vi "GEM_BANK_Add_Data.vi"(8 "error in (no error)":errorcluster, 10 "GEM_DATA":T1, 11 "LVBANK in":refnum<class "GEM_BANK.lvclass">) -> (0 "error out":errorcluster, 2 "Bank Size (bytes)":u32, 3 "LVBANK out":refnum<class "GEM_BANK.lvclass">)   [LabVIEW 2018, in "GEM_BANK.lvclass"]
uses:
  GEM_BANK.lvclass
  GEM_DATA_cluster_typedef.ctl
  GEM_BANK.lvclass/GEM_BANK.ctl
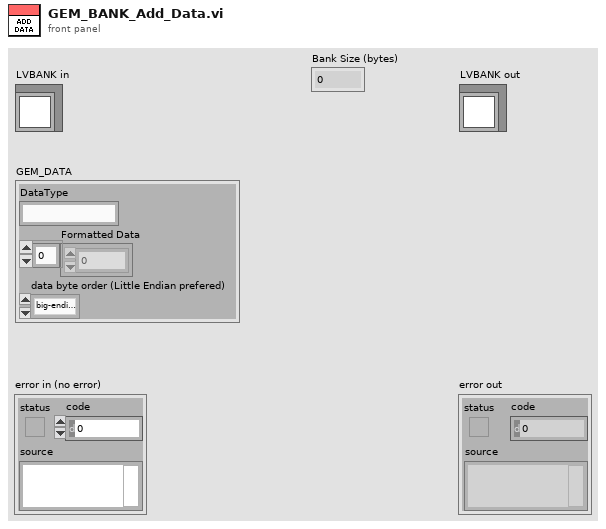
[diagram p1: front panel]
types:
  T1 = typedef "GEM_DATA_cluster_typedef.ctl" = cluster{"DataType":string, "Formatted Data":u8[], "data byte order (Little Endian prefered)":enum16{"big-endian, network order", "native, host order", "little-endian"}}
  T2 = enum16{"big-endian, network order", "native, host order", "little-endian"}
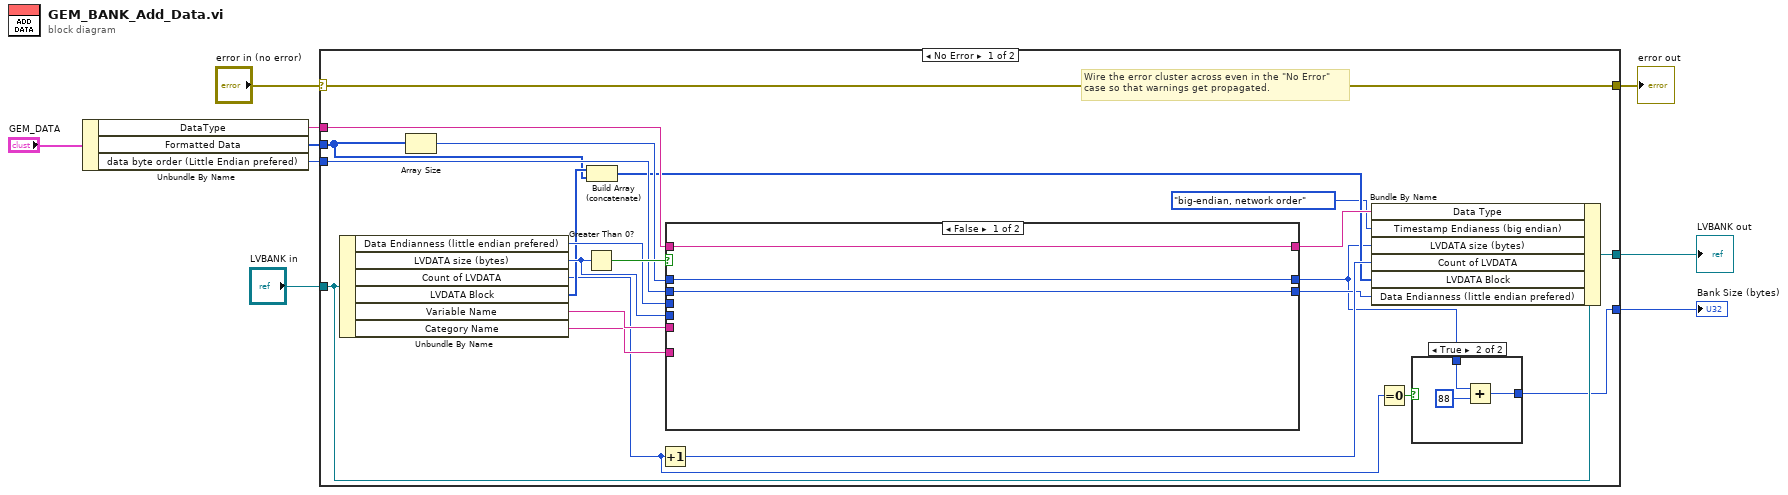
[diagram p0: block diagram]
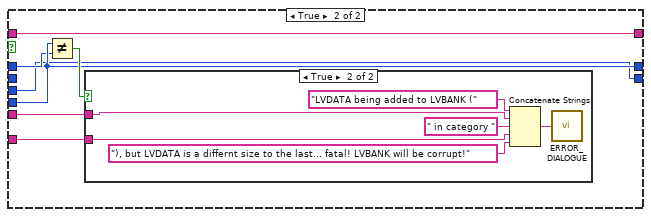
[diagram p3: hidden frame]
diagram:
  n1 = Unbundle By Name("GEM_DATA") -> ("DataType"=w3:string, "Formatted Data"=w4:u8[], "data byte order (Little Endian prefered)"=w2:T2)
  n2 = case shown="No Error" "error in (no error)" {
    selector: "error in (no error)" -> [w31 w53]
    tunnel: [w31 w53] -> w8
    tunnel: [w29 w52] -> w6
    tunnel: "LVBANK in" -> [w28 w52]
    tunnel: w2 -> [w25 _]
    tunnel: w3 -> [w23 _]
    tunnel: w4 -> [w18 _]
    tunnel: [w10 _] -> w1
    frame No Error {
      # "Wire the error cluster across even in the \"No Error\"\ncase so that warnings get propagated."
      n3 = Unbundle By Name(w28) -> ("Data Endianness (little endian prefered)"=w26:T2, "LVDATA size (bytes)"=w21:u32, "Count of LVDATA"=w12:i32, "LVDATA Block"=w20:u8[], "Variable Name"=w17:string, "Category Name"=w16:string)
      n4 = Array Size(array=w18) -> (size(s)=w22:i32)
      n5 = Greater Than 0?(x=w21) -> (x > 0?=w30:bool)
      n6 = Build Array (concatenate)(w20, w18) -> (w19:u8[])
      n7 = Increment(x=w12) -> (x+1=w27:i32)
      n8 = case shown="False" w30 {
        tunnel: [w38 w44] -> w11
        tunnel: w21 -> [_ w44]
        tunnel: w22 -> [w38 w43]
        tunnel: [w37 w42] -> w15
        tunnel: w26 -> [_ w42]
        tunnel: w25 -> [w37 _]
        tunnel: [w36 w41] -> w24
        tunnel: w23 -> [w36 w41]
        tunnel: w17 -> [_ w40]
        tunnel: w16 -> [_ w39]
        frame False {
        }
        frame True {
          n9 = Not Equal?(x=w44, y=w43) -> (x != y?=w45:bool)
          n10 = case shown="True" w45 {
            tunnel: w40 -> [_ w50]
            tunnel: w39 -> [_ w49]
            frame False {
            }
            frame True {
              n11 = Concatenate Strings("LVDATA being added to LVBANK (" ("string"), w50, " in category " ("string"), w49, "), but LVDATA is a differnt size to the last... fatal! LVBANK will be corrupt!" ("string")) -> (w46:string)
              n12 = call "ERROR_DIALOGUE.vi"("String"=w46) -> ()
            }
          }
        }
      }
      n13 = Bundle By Name(cluster=w28, "Data Type"=w24, "Timestamp Endianess (big endian)"=T2."big-endian, network order", "LVDATA size (bytes)"=w11, "Count of LVDATA"=w27, "LVDATA Block"=w19, "Data Endianness (little endian prefered)"=w15) -> (w29:refnum<class "GEM_BANK.lvclass">)
      n14 = Equal To 0?(x=w12) -> (x = 0?=w13:bool)
      n15 = case shown="True" w13 {
        tunnel: w11 -> [w32 w35]
        tunnel: [w32 w34] -> w10
        frame False {
        }
        frame True {
          n16 = Add(x=w35, y=u32 88) -> (x+y=w34:u32)
        }
      }
    }
    frame Error {
    }
  }
  "error out" <- w8
  "LVBANK out" <- w6
  "Bank Size (bytes)" <- w1
